vi "Show table lines.vi"(8 "error in":errorcluster, 10 "Show Table Lines":bool, 11 "AppendTable":refnum<k7>) -> (0 "error out":errorcluster)   [LabVIEW 2015, in "NI_ReportGenerationCore.lvlib"]
uses:
  <vilib>/Utility/NIReport.llb/NI_ReportGenerationCore.lvlib
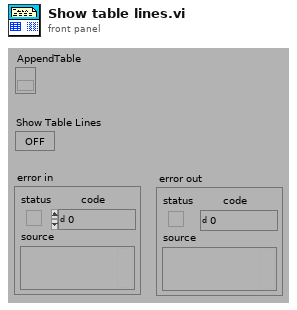
[diagram p1: front panel]
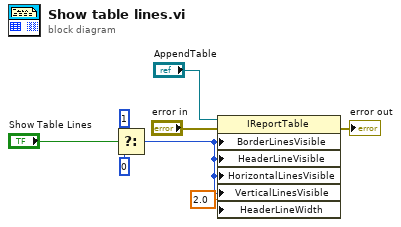
[diagram p0: block diagram]
diagram:
  n1 = Select(t=1 ("BorderLinesVisible"), s="Show Table Lines", f=0 ("BorderLinesVisible")) -> (s? t:f=w4:i32)
  n2 = property class="IReportTable"(reference="AppendTable", error in="error in", "BorderLinesVisible"=w4, "HeaderLineVisible"=w4, "HorizontalLinesVisible"=w4, "VerticalLinesVisible"=w4, "HeaderLineWidth"=2.0) -> (error out=→"error out":errorcluster)  [unwired: 1 out]
